vi "DisconnectSW.vi"(6 "Legacy (f)?":bool, 8 "error in (no error)":errorcluster, 10 "SW Device Name":string) -> (0 "error out":errorcluster)   [LabVIEW 2011]
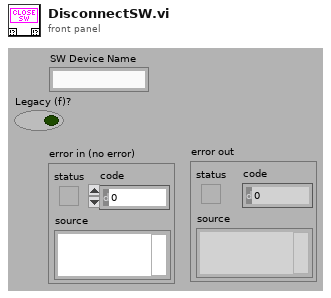
[diagram p1: front panel]
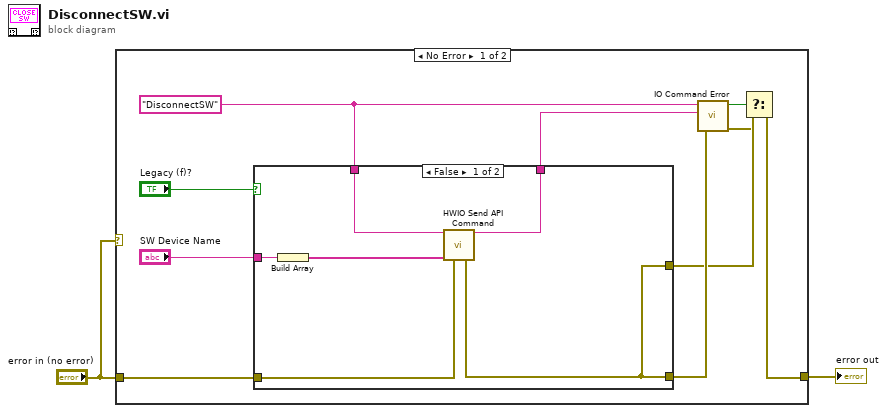
[diagram p0: block diagram]
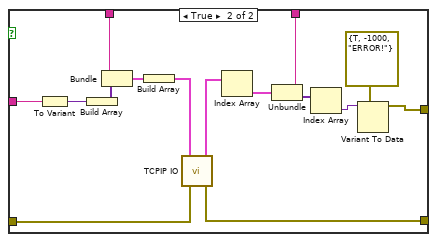
[diagram p2: hidden frame]
diagram:
  n1 = case shown="No Error" "error in (no error)" {
    tunnel: "error in (no error)" -> [w12 w34]
    tunnel: [w5 w34] -> w2
    frame No Error {
      w10 = "DisconnectSW"
      n2 = case shown="False" "Legacy (f)?" {
        tunnel: w12 -> [w18 w33]
        tunnel: [w17 w31] -> w11
        tunnel: w10 -> [w15 w30]
        tunnel: [w16 w29] -> w9
        tunnel: [w17 w22] -> w7
        tunnel: "SW Device Name" -> [w14 w19]
        frame False {
          n3 = Build Array(w14) -> (w13:string[])
          n4 = call "HWIO Send API Command.vi"("Action"=w15, "String"=w13, "error in (no error)"=w18) -> ("Action out"=w16:string, "error out"=w17:errorcluster)  [unwired: 5 in, 6 out]
        }
        frame True {
          n5 = To Variant(anything=w19) -> (Variant=w21:variant)
          n6 = Build Array(w21) -> (w20:variant[])
          n7 = Bundle(w30, w20) -> (w32:cluster{string, variant[]})  [unwired: 1 out]
          n8 = Build Array(w32) -> (w28:cluster{string, variant[]}[])
          n9 = call "TCPIP IO.vi"("error in (no error)"=w33, "Commands"=w28) -> ("error out"=w31:errorcluster, "Responses"=w26:cluster{string, variant[]}[])  [unwired: 1 in, 3 out]
          n10 = Index Array(array=w26) -> (element=w27:cluster{string, variant[]})  [unwired: 1 in]
          n11 = Unbundle(w27) -> (w29:string, w25:variant[])
          n12 = Index Array(array=w25) -> (element=w24:variant)  [unwired: 1 in]
          n13 = Variant To Data(type=errorcluster {"status"=TRUE, "code"=-1000, "source"="ERROR!"} ("error out"), Variant=w24) -> (data=w22:errorcluster)  [unwired: 1 in, 1 out]
        }
      }
      n14 = call "IO Command Error.vi"("error in (no error)"=w11, "Command Returned (\"\")"=w9, "Command Sent (\"\")"=w10) -> ("error out"=w6:errorcluster, "HW ERR?"=w8:bool)  [unwired: 3 out]
      n15 = Select(t=w7, s=w8, f=w6) -> (s? t:f=w5:errorcluster)
    }
    frame Error {
    }
  }
  "error out" <- w2
